vi "startHW.vi"(8 "error in (no error)":errorcluster, 11 "CompactRIO in":refnum<class "CompactRIO.lvclass">) -> (0 "error out":errorcluster, 3 "CompactRIO out":refnum<class "CompactRIO.lvclass">)   [LabVIEW 2015, in "CompactRIO.lvclass"]
doc: "Performs any operations necessary to start the hardware. For a cRIO target on first call it starts the FPGA VI, generating a user event with the FPGA VI reference for use elsewhere, configures the interrupt behavior, and allots some time to allow the FPGA to start updating properly."
uses:
  CompactRIO.lvclass
  CompactRIO.lvclass/CompactRIO.ctl
  ComponentTemplateCore/ComponentModel/ComponentModelRT/ConfigurationHandler/RIOConfig/RIOConfig.lvclass/RIOConfig.ctl
  ComponentTemplateCore/ComponentModel/ComponentModelRT/ConfigurationHandler/IRQConfig/IRQConfig.lvclass/IRQConfig.ctl
  <vilib>/FPGAPlugInAG/cRIO-9074/niLvFpga_Open_cRIO-9074.vi
  <vilib>/FPGAPlugInAG/cRIO-9074/niLvFpga_Run_cRIO-9074.vi
  <vilib>/Utility/error.llb/Error Cluster From Error Code.vi
  <vilib>/rvi/errors/niLvFpgaAdjustHostInterfaceError.vi
  <vilib>/RVI Host/nirviSupport.llb/nirviErrorClusterFromErrorCode.vi
  ComponentTemplateCore/ComponentModel/ComponentModelRT/RIOHandler/IRIOHandler/IRIOHandler.lvclass
  <vilib>/rvi/interface/nirviOpenFPGA/nirviOpenFPGA.xnode
  fpgaVIReference.ctl
  FPGA Bitfiles/cRIOApp_FPGATarget_fpgaMain_F827BADB.lvbitx
  <vilib>/rvi/interface/nirviUpCast/nirviUpCast.xnode
  <vilib>/rvi/interface/nirviMethod/nirviMethod.xnode
  ComponentTemplateCore/ComponentModel/ComponentModelRT/Typedefs/FPGAVIRefCRIO9074.ctl
  <vilib>/rvi/interface/nirviReadWriteControl/nirviReadWriteControl.xnode
  ComponentTemplateCore/ComponentModel/ComponentModelRT/LoopTimer/ILoopTimer/ILoopTimer.lvclass
  ComponentTemplateCore/ComponentModel/ComponentModelRT/IRQHandler/IIRQHandler/IIRQHandler.lvclass
  ComponentTemplateCore/ComponentModel/ComponentModelRT/ConfigurationHandler/RIOConfig/RIOConfig.lvclass
  ComponentTemplateCore/ComponentModel/ComponentModelRT/ConfigurationHandler/IRQConfig/IRQConfig.lvclass
  <vilib>/rvi/interface/nirviMethod/StockFPGA_InlinedMethodWaitForSingleIRQ.vi
  <vilib>/FPGAPlugInAG/cRIO-9074/niLvFpga_WaitOnIrq_cRIO-9074.vi
  NiFpgaLv.dll
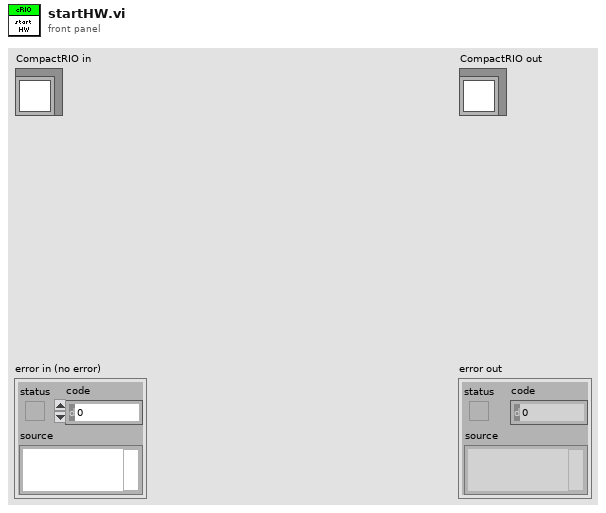
[diagram p1: front panel]
types:
  T1 = typedef "fpgaVIReference.ctl" = refnum<k20>
  T2 = typedef "fpgaVIRefCRIO9074.ctl" = refnum<k20>
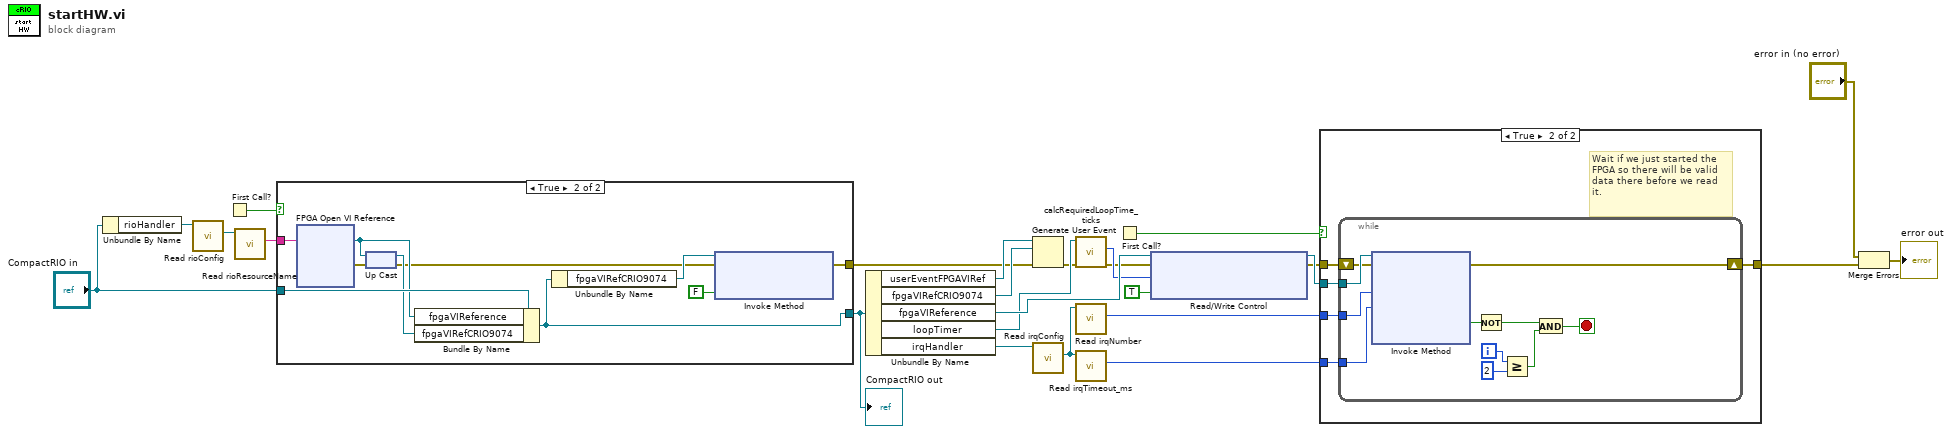
[diagram p0: block diagram]
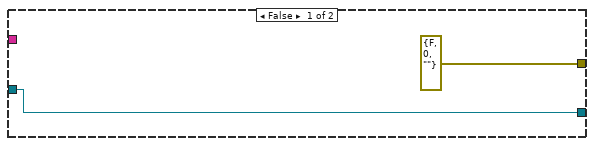
[diagram p3: hidden frame]
diagram:
  n1 = Unbundle By Name("CompactRIO in") -> ("rioHandler"=w22:refnum<class "IRIOHandler.lvclass">)
  n2 = call-dynamic "Read rioConfig.vi"("IRIOHandler in"=w22) -> ("RIOConfig.lvclass"=w23:refnum<class "RIOConfig.lvclass">)  [unwired: 8 in, 2 out]
  n3 = First Call?() -> (First Call?: T/F=w24:bool)
  n4 = call "Read rioResourceName.vi"("RIOConfig in"=w23) -> ("rioResourceName"=w25:string)  [unwired: 8 in, 2 out]
  n5 = case shown="True" w24 {
    tunnel: [w27 w32] -> w12
    tunnel: w25 -> [_ w37]
    tunnel: [errorcluster {"status"=FALSE, "code"=0, "source"=""} ("error out") w28] -> w2
    tunnel: "CompactRIO in" -> [w27 w35]
    frame False {
    }
    frame True {
      n6 = xnode "FPGA Open VI Reference"("resource name"=w37) -> ("FPGA VI Reference Out"=w33:T1, "error out"=w36:errorcluster)  [unwired: 1 in]
      n7 = xnode "Up Cast"("FPGA VI Reference In"=w33, "error in"=w36) -> ("FPGA VI Reference Out"=w34:refnum<k20>, "error out"=w29:errorcluster)
      n8 = Bundle By Name(cluster=w35, "fpgaVIReference"=w33, "fpgaVIRefCRIO9074"=w34) -> (w32:refnum<class "CompactRIO.lvclass">)
      n9 = Unbundle By Name(w32) -> ("fpgaVIRefCRIO9074"=w31:T2)
      n10 = xnode "Invoke Method"("FPGA VI Reference In"=w31, "error in"=w29, "Wait Until Done (F)"=FALSE) -> ("error out"=w28:errorcluster)  [unwired: 1 out]
    }
  }
  "CompactRIO out" <- w12
  n11 = Unbundle By Name(w12) -> ("userEventFPGAVIRef"=w4:refnum<user-event>, "fpgaVIRefCRIO9074"=w3:T2, "fpgaVIReference"=w21:T1, "loopTimer"=w19:refnum<class "ILoopTimer.lvclass">, "irqHandler"=w8:refnum<class "IIRQHandler.lvclass">)
  n12 = Generate User Event(user event=w4, event data cluster=w3, error in=w2) -> (error out=w1:errorcluster)  [unwired: 1 in, 1 out]
  n13 = call-dynamic "Read irqConfig.vi"("IIRQHandler in"=w8) -> ("irqConfig"=w5:refnum<class "IRQConfig.lvclass">)  [unwired: 8 in, 2 out]
  n14 = call-dynamic "calcRequiredLoopTime_ticks.vi"("error in (no error)"=w1, "ILoopTimer in"=w19) -> ("error out"=w15:errorcluster, "requiredLoopTime_ticks"=w16:u32)  [unwired: 6 in, 2 out]
  n15 = call "Read irqNumber.vi"("IRQConfig in"=w5) -> ("irqNumber"=w7:i32)  [unwired: 8 in, 2 out]
  n16 = call "Read irqTimeout_ms.vi"("IRQConfig in"=w5) -> ("irqTimeout_ms"=w6:i32)  [unwired: 8 in, 2 out]
  n17 = First Call?() -> (First Call?: T/F=w18:bool)
  n18 = xnode "Read/Write Control"("FPGA VI Reference In"=w21, "error in"=w15, "loopPeriod_ticks"=w16, "waitUntilIRQClearedIsTrue"=TRUE ("Wait Until Cleared")) -> ("FPGA VI Reference Out"=w17:T1, "error out"=w14:errorcluster)
  n19 = case shown="True" w18 {
    tunnel: w17 -> [_ w50]
    tunnel: w14 -> [w45 w49]
    tunnel: [w45 w48] -> w10
    tunnel: w7 -> [_ w47]
    tunnel: w6 -> [_ w46]
    frame False {
    }
    frame True {
      # "Wait if we just started the  FPGA so there will be valid data there before we read it."
      n20 = while {
        tunnel: w50 -> [w61]
        shift-right: [w54] -> w48
        shift-left: w49 -> [w55]
        tunnel: w47 -> [w52]
        tunnel: w46 -> [w51]
        i -> [w53]
        stop <- w56 stop-if-true
        n21 = xnode "Invoke Method"("FPGA VI Reference In"=w61, "error in"=w55, "IRQ Number(s)"=w52, "Timeout (ms)"=w51) -> ("error out"=w54:errorcluster, "Timed Out"=w57:bool)  [unwired: 2 out]
        n22 = Not(x=w57) -> (.not. x?=w59:bool)
        n23 = Greater Or Equal?(x=w53, y=2) -> (x >= y?=w58:bool)
        n24 = And(x=w59, y=w58) -> (x .and. y?=w56:bool)
      }
    }
  }
  n25 = Merge Errors("error in (no error)", w10) -> (→"error out":errorcluster)
